vi "time1.vi"() -> ()   [LabVIEW 2020]
panel:
  out "time 1":T1
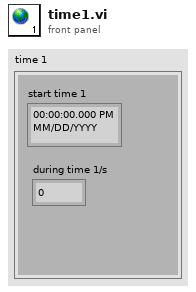
[diagram p1: front panel]
types:
  T1 = cluster{"start time 1":timestamp, "during time 1/s":dbl}
diagram:
